vi "Test_StartMessageCycle_Wait_MultipleReceived.vi"(8 "error in (no error)":errorcluster, 11 "TestCase in":refnum<class "TestMessageCycle.lvclass">) -> (0 "error out":errorcluster, 3 "TestCase out":refnum<class "TestMessageCycle.lvclass">)   [LabVIEW 2017, in "TestMessageCycle.lvclass"]
uses:
  TestMessageCycle.lvclass
  <vilib>/ActorFramework/Message/Message.lvclass
  Source/MessageCycle/MessageCycle.lvclass/MessageCycle.ctl
  <vilib>/ActorFramework/Message Enqueuer/Message Enqueuer.lvclass/Message Enqueuer.ctl
  01b4bbe5-fd6e-4a3f-b032-985426bfee4c.vi
  <vilib>/ActorFramework/Message Enqueuer/Enqueue.vi
  Doubles/ActorCountsMessageCycles/ActorCountsMessageCycles.lvclass
  C:/Program Files (x86)/National Instruments/LabVIEW 2017/vi.lib/ActorFramework/Actor/Actor.lvclass
  Source/MessageCycle/MessageCycle.lvclass
  C:/Program Files (x86)/National Instruments/LabVIEW 2017/vi.lib/ActorFramework/Message/Message.lvclass
  <vilib>/ActorFramework/Stop Msg/Stop Msg.lvclass
  Source/MessageCycle/Launch Deferred Timeout Notifier.vi
  <vilib>/ActorFramework/Message Priority Queue/Priority Enqueue.vi
  <vilib>/ActorFramework/Actor/Actor.lvclass
panel:
  out "Cyclic Messages Received":u32
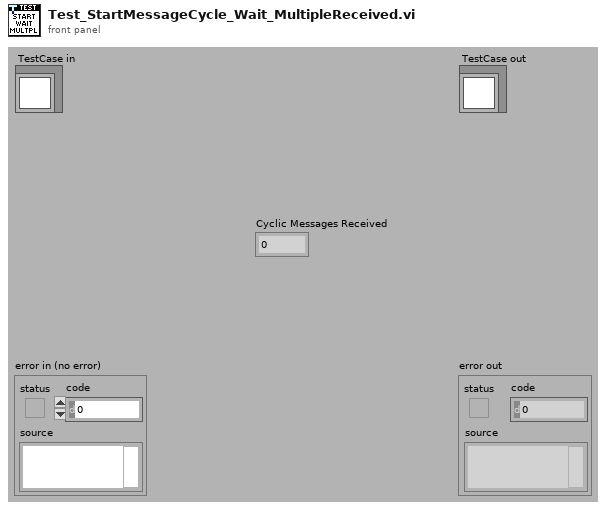
[diagram p1: front panel]
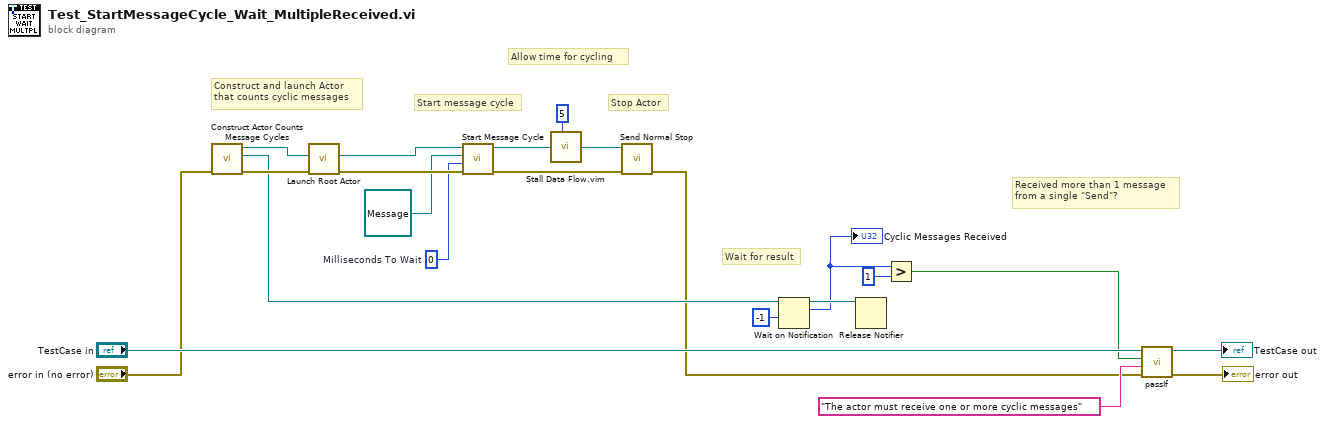
[diagram p0: block diagram]
diagram:
  w18 = 0  # Milliseconds To Wait
  # "Allow time for cycling"
  # "Wait for result"
  # "Stop Actor"
  # "Start message cycle"
  # "Received more than 1 message\nfrom a single \"Send\"?"
  # "Construct and launch Actor\nthat counts cyclic messages"
  n1 = call "Construct Actor Counts Message Cycles.vi"("error in (no error)"="error in (no error)") -> ("error out"=w10:errorcluster, "Final Count"=w9:refnum<notifier>, "ActorCountsMessageCycles"=w12:refnum<class "ActorCountsMessageCycles.lvclass">)  [unwired: 8 in]
  n2 = call <vilib>:"Launch Root Actor.vi"("error in (no error)"=w10, "Actor"=w12) -> ("error out"=w22:errorcluster, "Actor's Enqueuer"=w16:refnum<class "Message Enqueuer.lvclass">)  [unwired: 8 in]
  n3 = call "Start Message Cycle.vi"("error in (no error)"=w22, "Inter-Message Wait [ms] (0)"=w18, "Message"=refnum<class "Message.lvclass"> refnum, "Message Enqueuer"=w16) -> ("error out"=w17:errorcluster, "Message Enqueuer out"=w15:refnum<class "Message Enqueuer.lvclass">)  [unwired: 5 in, 1 out]
  n4 = call "Stall Data Flow.vim"("value in"=w15, "milliseconds to wait"=u32 5) -> ("value out"=w5:refnum<class "Message Enqueuer.lvclass">)  [unwired: 1 out]
  n5 = call <vilib>:"Send Normal Stop.vi"("error in (no error)"=w17, "Message Enqueuer"=w5) -> ("error out"=w6:errorcluster)  [unwired: 9 in]
  n6 = Wait on Notification(notifier=w9, timeout in ms (-1)=-1) -> (notifier out=w7:refnum<notifier>, notification=w3:u32)  [unwired: 2 in, 2 out]
  "Cyclic Messages Received" <- w3
  n7 = Release Notifier(notifier=w7) -> ()  [unwired: 2 in, 3 out]
  n8 = Greater?(x=w3, y=u32 1) -> (0:w14:bool)
  n9 = call-dynamic "passIf.vi"("error in (no error)"=w6, "message (\"\")"="The actor must receive one or more cyclic messages" ("message (\"\")"), "pass"=w14, "TestCase in"="TestCase in") -> ("error out"=→"error out":errorcluster, "TestCase out"=→"TestCase out":refnum<class "TestMessageCycle.lvclass">)  [unwired: 6 in]
